vi "StopProg.vi"(11 "Stop (f)":bool) -> (3 "Stop?":bool)   [LabVIEW 2017, in "Framework.lvlib"]
uses:
  Framework.lvlib
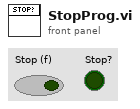
[diagram p1: front panel]
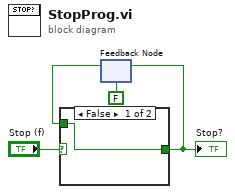
[diagram p0: block diagram]
diagram:
  n1 = feedback #1(FALSE) -> (w1:bool)
  n2 = case shown="False" "Stop (f)" {
    selector: "Stop (f)" -> [_ w6]
    tunnel: [w5 w6] -> w3
    tunnel: w1 -> [w5 _]
    frame False {
    }
    frame True {
    }
  }
  "Stop?" <- w3
  n3 = feedback-in #1(w3) -> ()
